vi "Configure IO Control.vi"(6 "Mode":u8=1 min=1 format="%.0x", 8 "error in (no error)":errorcluster, 9 "ID":u16=1 min=1 format="%.0x", 10 "Existing PIDs":string[](array[string]), 11 "Name":string) -> (0 "error out":errorcluster, 1 "ID out":u16, 2 "Cancel PID?":bool, 3 "Name out":string, 4 "Mode out":u8)   [LabVIEW 2015, in "Diagnostics Addon System Explorer.lvlib"]
uses:
  Diagnostics Addon System Explorer.lvlib
  <vilib>/NI/AMC/Create Single Message.vi
  <vilib>/NI/AMC/Update Message Routing Info.vi
  <vilib>/NI/AMC/Read Termination Message.vi
  <vilib>/NI/AMC/Send Message.vi
  <vilib>/NI/AMC/Globals.vi
  <vilib>/NI/AMC/AMC.lvlib
panel:
  in  "Cancel PID":bool
  in  "Apply":bool
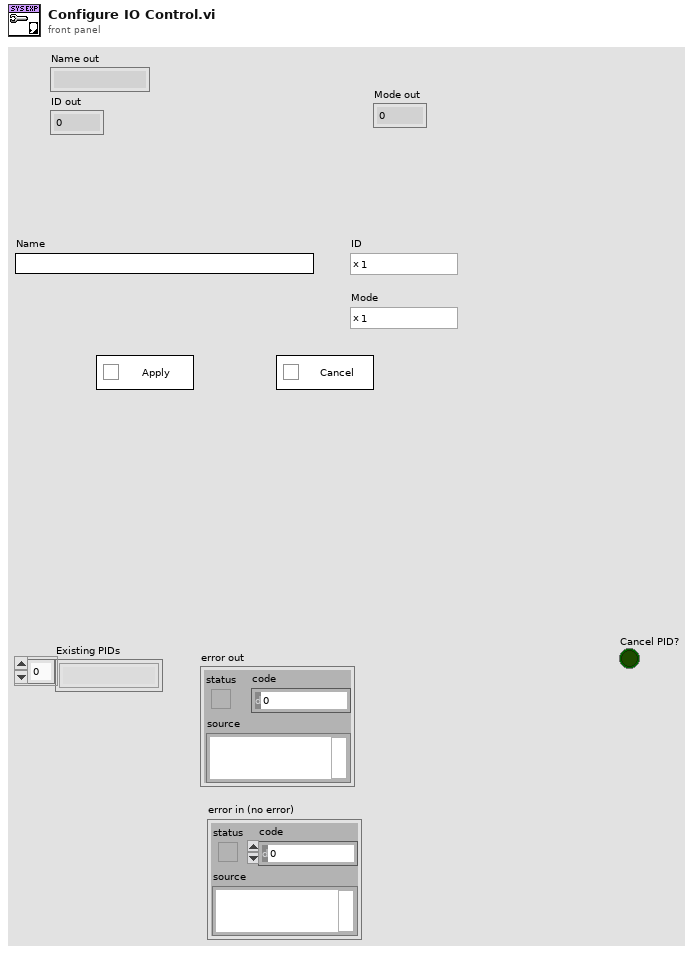
[diagram p1: front panel]
types:
  T1 = cluster{"Apply":refnum<vi>, "Cancel PID":refnum<vi>}
  T2 = typedef "AMC.lvlib/Message Queue.ctl" = refnum<queue>
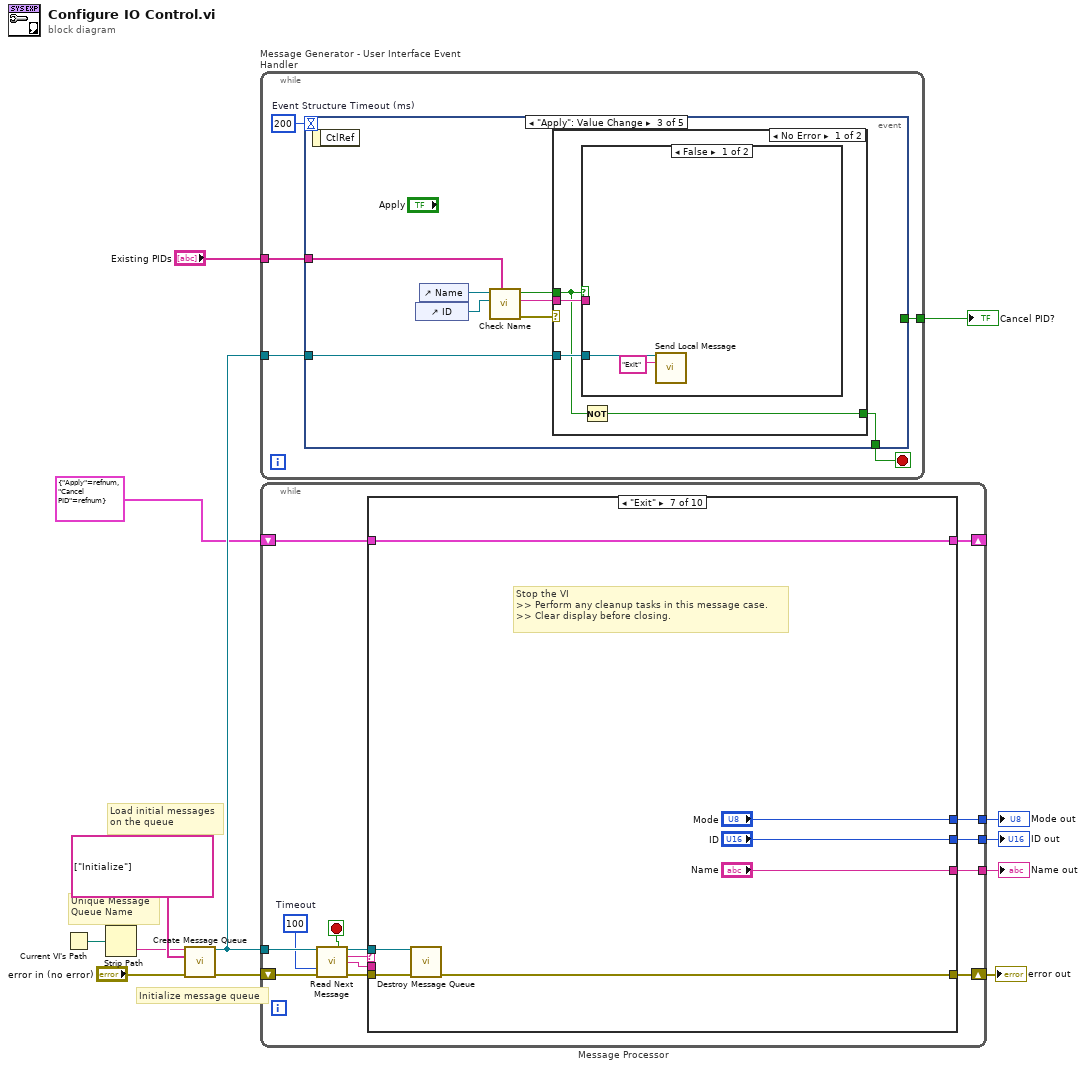
[diagram p0: block diagram]
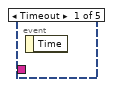
[diagram p2: hidden frame]
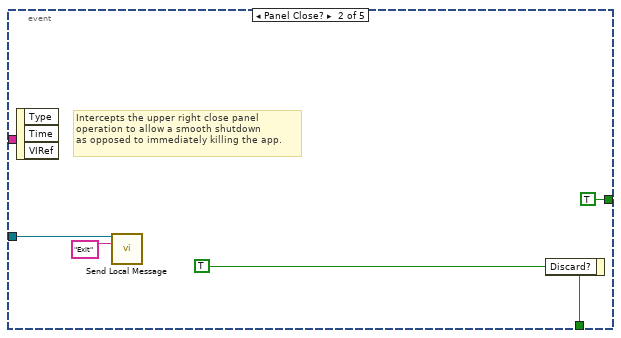
[diagram p3: hidden frame]
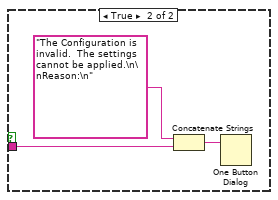
[diagram p4: hidden frame]
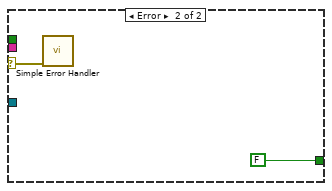
[diagram p5: hidden frame]
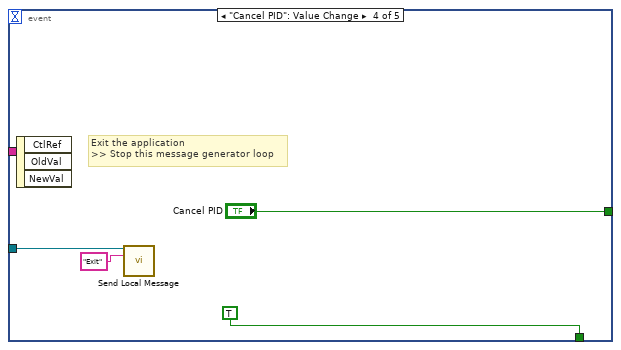
[diagram p6: hidden frame]
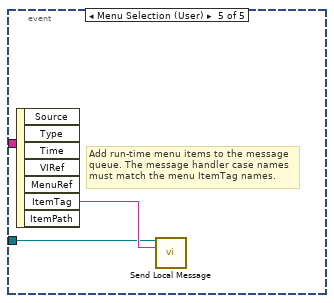
[diagram p7: hidden frame]
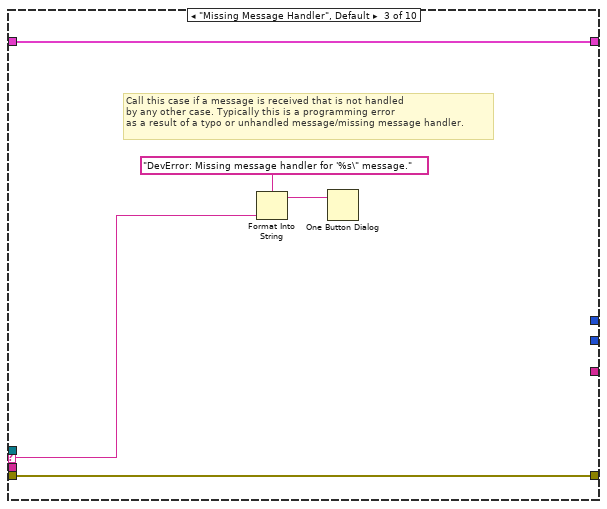
[diagram p10: hidden frame]
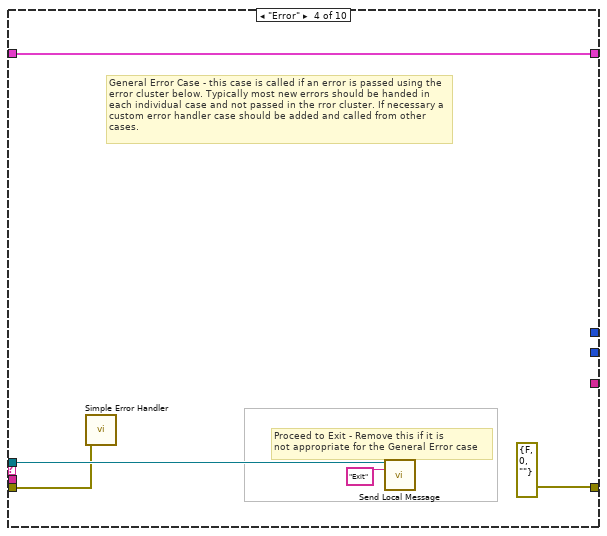
[diagram p11: hidden frame]
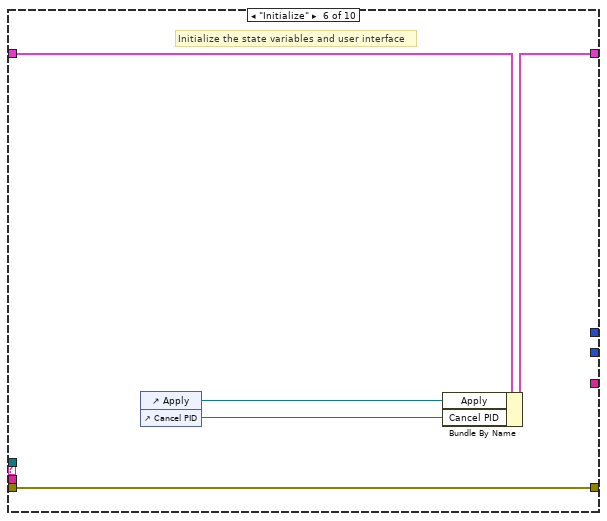
[diagram p13: hidden frame]
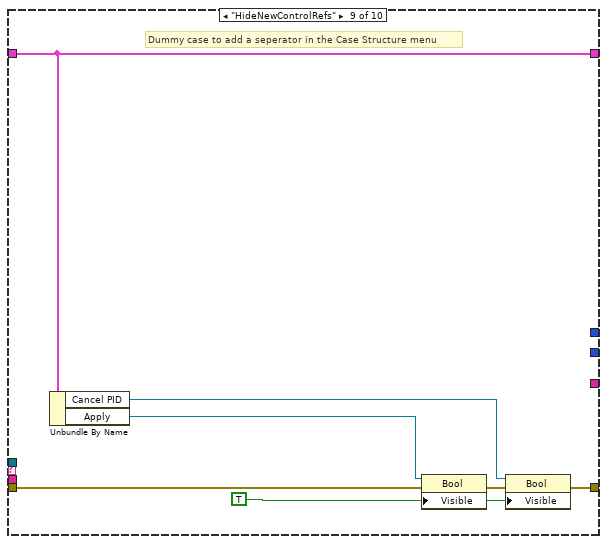
[diagram p15: hidden frame]
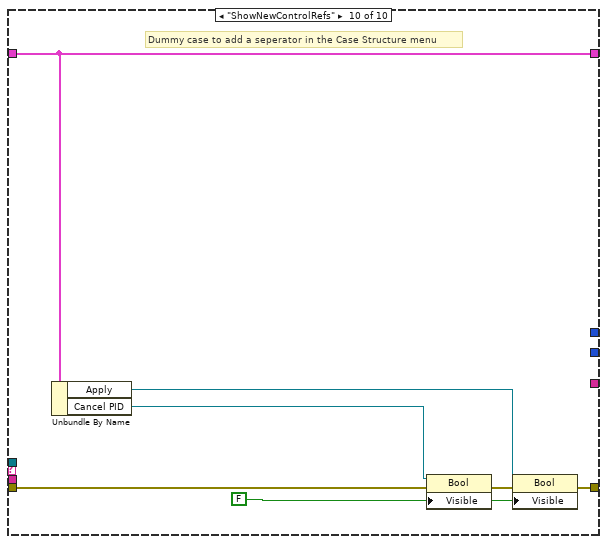
[diagram p16: hidden frame]
diagram:
  # "Initialize message queue"
  # "Unique Message\nQueue Name"
  # "Load initial messages\non the queue"
  n1 = Current VI's Path() -> (path=w9:path)
  n2 = Strip Path(path=w9) -> (name=w12:string)  [unwired: 1 out]
  n3 = call <vilib>:"Create Message Queue.vi"("message queue name"=w12, "initial message names"=string[] ["Initialize"], "error in"="error in (no error)") -> ("message queue out"=w11:T2, "error out"=w10:errorcluster)  [unwired: 11 in]
  n4 = while "Message Generator - User Interface Event Handler" {
    tunnel: w11 -> [w16]
    tunnel: [w15] -> w7
    tunnel: "Existing PIDs" -> [w14]
    stop <- w17 stop-if-true
    w18 = 200  # Event Structure Timeout (ms)
    n5 = event shown="[2] \"Apply\": Value Change" {
      selector: _ -> [_ _ _ _ _]
      dyn-events: _ -> [_ _ _ _ _]
      timeout: w18 -> [_ _ _ _ _]
      tunnel: [_ w22 w29 TRUE ("Discard?") _] -> w17
      tunnel: w16 -> [_ w20 w30 w43 w46]
      tunnel: [_ TRUE ("Cancel PID") _ "Cancel PID" _] -> w15
      tunnel: w14 -> [_ _ w23 _ _]
      event Timeout {
        n6 = event-data() -> ()  [unwired: 2 out]
      }
      event Panel Close? {
        w22 = TRUE ("Discard?")
        # "Intercepts the upper right close panel\noperation to allow a smooth shutdown\nas opposed to immediately killing the app."
        n7 = event-data() -> ()  [unwired: 4 out]
        n8 = call <vilib>:"Send Local Message.vi"("message queue in"=w20, "message name"="Exit") -> ()  [unwired: 11 in, 3 out]
        n9 = event-data("Discard?"=w22) -> ()  [unwired: 1 in, 1 out]
      }
      event "Apply": Value Change {
        n10 = event-data() -> ()  [unwired: 2 out]
        n11 = control-ref of="ID"() -> (w25:refnum<vi>)
        n12 = control-ref of="Name"() -> (w24:refnum<vi>)
        n13 = call "Check Name.vi"("Existing PIDs"=w23, "ID"=w25, "Name"=w24) -> ("error out"=w28:errorcluster, "String"=w26:string, "Boolean"=w27:bool)  [unwired: 6 in]
        n14 = case shown="No Error" w28 {
          selector: w28 -> [_ w41]
          tunnel: w27 -> [w32 _]
          tunnel: w30 -> [w34 _]
          tunnel: w26 -> [w33 _]
          tunnel: [w31 FALSE] -> w29
          frame No Error {
            n15 = case shown="False" w32 {
              tunnel: w34 -> [w36 _]
              tunnel: w33 -> [_ w39]
              frame False {
                n16 = call <vilib>:"Send Local Message.vi"("message queue in"=w36, "message name"="Exit" ("Message Name")) -> ()  [unwired: 11 in, 3 out]
              }
              frame True {
                n17 = Concatenate Strings("The Configuration is invalid.  The settings cannot be applied.\n\nReason:\n" ("message"), w39) -> (w37:string)
                n18 = One Button Dialog(message=w37) -> ()  [unwired: 1 in, 1 out]
              }
            }
            n19 = Not(x=w32) -> (.not. x?=w31:bool)
          }
          frame Error {
            n20 = call <vilib>:"Simple Error Handler.vi"("error in (no error)"=w41) -> ()  [unwired: 4 in, 5 out]
          }
        }
      }
      event "Cancel PID": Value Change {
        # "Exit the application\n>> Stop this message generator loop"
        n21 = event-data() -> ()  [unwired: 4 out]
        n22 = call <vilib>:"Send Local Message.vi"("message queue in"=w43, "message name"="Exit") -> ()  [unwired: 11 in, 3 out]
      }
      event Menu Selection (User) {
        # "Add run-time menu items to the message\nqueue. The message handler case names must match the menu ItemTag names."
        n23 = event-data() -> ("ItemTag"=w47:string)  [unwired: 7 out]
        n24 = call <vilib>:"Send Local Message.vi"("message queue in"=w46, "message name"=w47) -> ()  [unwired: 11 in, 3 out]
      }
    }
  }
  "Cancel PID?" <- w7
  n25 = while "Message Processor" {
    shift-left: w10 -> [w55]
    shift-right: [w59] -> w5
    tunnel: w11 -> [w56]
    shift-left: T1 {"Apply"=refnum, "Cancel PID"=refnum} ("State Variables") -> [w61]
    shift-right: [w60] -> _
    tunnel: [w50] -> w3
    tunnel: [w49] -> w2
    tunnel: [w48] -> w1
    stop <- w58 stop-if-true
    w53 = 100  # Timeout
    n26 = call <vilib>:"Read Next Message.vi"("message queue in"=w56, "timeout (1 ms)"=w53, "error in"=w55) -> ("exit process?"=w58:bool, "message queue out"=w57:T2, "message name"=w52:string, "message value"=w51:string, "error out"=w54:errorcluster)  [unwired: 5 in, 3 out]
    n27 = case shown="\"Exit\"" w52 {
      selector: w52 -> [_ _ w68 _ _ _ _ _ _ _]
      tunnel: [w63 w65 w70 w75 w77 w81 w87 w91 w98 w105] -> w60
      tunnel: w61 -> [w63 w65 w70 w75 w77 w82 w87 w91 w98 w105]
      tunnel: w57 -> [_ _ _ w73 _ _ w88 _ _ _]
      tunnel: w54 -> [w62 w64 w69 w71 w76 w80 w89 w90 w92 w99]
      tunnel: [w62 w64 w69 errorcluster {"status"=FALSE, "code"=0, "source"=""} ("error out") w76 w80 w86 w90 w95 w103] -> w59
      tunnel: w51 -> [_ _ _ _ _ _ _ _ _ _]
      tunnel: [_ _ _ _ _ _ "Name" _ _ _] -> w50
      tunnel: [_ _ _ _ _ _ "ID" _ _ _] -> w49
      tunnel: [_ _ _ _ _ _ "Mode" _ _ _] -> w48
      frame "---------- Framework Operations ----------" {
        # "Dummy case to add a seperator in the Case Structure menu"
      }
      frame "", "Idle" {
        # "Idle Case - this case is called after a Timeout on the Get Next Message from Queue VI, if no new messages are present on the queue. This case can be used for housekeeping tasks such as updating the UI."
      }
      frame "Missing Message Handler", Default {
        # "Call this case if a message is received that is not handled \nby any other case. Typically this is a programming error\nas a result of a typo or unhandled message/missing message handler."
        n28 = Format Into String(format string="DevError: Missing message handler for '%s\" message." ("message"), w68) -> (resulting string=w66:string)  [unwired: 2 in, 1 out]
        n29 = One Button Dialog(message=w66) -> ()  [unwired: 2 out]
      }
      frame "Error" {
        # "Proceed to Exit - Remove this if it is\nnot appropriate for the General Error case"
        # "General Error Case - this case is called if an error is passed using the error cluster below. Typically most new errors should be handed in each individual case and not passed in the rror cluster. If necessary a custom error handler case should be added and called from other cases."
        n30 = call <vilib>:"Simple Error Handler.vi"("error in (no error)"=w71) -> ()  [unwired: 1 in, 8 out]
        n31 = call <vilib>:"Send Local Message.vi"("message queue in"=w73, "message name"="Exit") -> ()  [unwired: 11 in, 3 out]
      }
      frame "---------- Generic Operations ----------" {
        # "Dummy case to add a seperator in the Case Structure menu"
      }
      frame "Initialize" {
        # "Initialize the state variables and user interface"
        n32 = control-ref of="Apply"() -> (w79:refnum<vi>)
        n33 = control-ref of="Cancel PID"() -> (w78:refnum<vi>)
        n34 = Bundle By Name(cluster=w82, "Apply"=w79, "Cancel PID"=w78) -> (w81:T1)
      }
      frame "Exit" {
        # "Stop the VI\n>> Perform any cleanup tasks in this message case.\n>> Clear display before closing."
        n35 = call <vilib>:"Destroy Message Queue.vi"("message queue in"=w88, "error in"=w89) -> ("error out"=w86:errorcluster)  [unwired: 11 in, 2 out]
      }
      frame "---------- Application Operations ----------" {
        # "Dummy case to add a seperator in the Case Structure menu"
      }
      frame "HideNewControlRefs" {
        w96 = TRUE ("Visible")
        # "Dummy case to add a seperator in the Case Structure menu"
        n36 = Unbundle By Name(w98) -> ("Cancel PID"=w93:refnum<vi>, "Apply"=w94:refnum<vi>)
        n37 = property class="Bool"(reference=w94, error in=w92, "Visible"=w96) -> (error out=w97:errorcluster)  [unwired: 1 out]
        n38 = property class="Bool"(reference=w93, error in=w97, "Visible"=w96) -> (error out=w95:errorcluster)  [unwired: 1 out]
      }
      frame "ShowNewControlRefs" {
        w102 = FALSE ("Visible")
        # "Dummy case to add a seperator in the Case Structure menu"
        n39 = Unbundle By Name(w105) -> ("Apply"=w101:refnum<vi>, "Cancel PID"=w100:refnum<vi>)
        n40 = property class="Bool"(reference=w100, error in=w99, "Visible"=w102) -> (error out=w104:errorcluster)  [unwired: 1 out]
        n41 = property class="Bool"(reference=w101, error in=w104, "Visible"=w102) -> (error out=w103:errorcluster)  [unwired: 1 out]
      }
    }
  }
  "error out" <- w5
  "Name out" <- w3
  "ID out" <- w2
  "Mode out" <- w1
